vi "Acquire Finite Frames.vi"(8 "error in (no error)":errorcluster, 11 "TroSpec in":refnum<class "PL ISTEQ TroSpec.lvclass">) -> (0 "error out":errorcluster, 1 "lost frames":u16, 2 "frame":u32[][](array[numeric]), 3 "TroSpec out":refnum<class "PL ISTEQ TroSpec.lvclass">)   [LabVIEW 2015, in "PL ISTEQ TroSpec.lvclass"]
doc: "Starts acquisition and reads the configured finite number of frames."
uses:
  PL ISTEQ TroSpec.lvclass
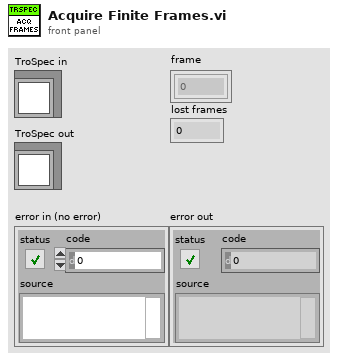
[diagram p1: front panel]
types:
  T1 = cluster{"period, s":dbl, "gain":u16, "offset":u16, "mode":cluster{"acquisition":bool, "service mode":bool, "inverted X":bool, "continuous acquisition":bool, "multiple exposures":bool}, "number of frames":u32, "exposure":u32}
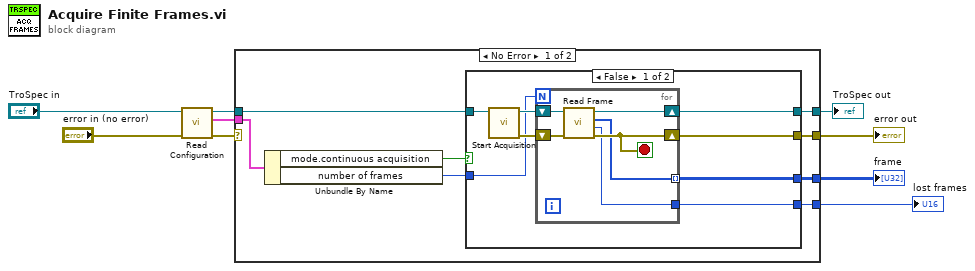
[diagram p0: block diagram]
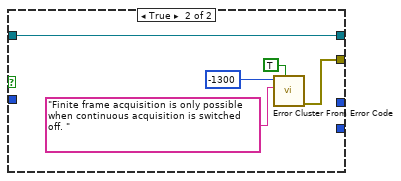
[diagram p2: hidden frame]
diagram:
  n1 = call "Read Configuration.vi"("error in (no error)"="error in (no error)", "TroSpec in"="TroSpec in") -> ("error out"=w7:errorcluster, "configuration"=w3:T1, "TroSpec out"=w6:refnum<class "PL ISTEQ TroSpec.lvclass">)  [unwired: 7 in]
  n2 = case shown="No Error" w7 {
    selector: w7 -> [_ w37]
    tunnel: w6 -> [w14 w38]
    tunnel: [w13 w38] -> w5
    tunnel: [w15 w37] -> w4
    tunnel: w3 -> [w17 _]
    tunnel: [w12 _] -> w2
    tunnel: [w11 _] -> w1
    frame No Error {
      n3 = Unbundle By Name(w17) -> ("mode.continuous acquisition"=w16:bool, "number of frames"=w10:u32)
      n4 = case shown="False" w16 {
        tunnel: [w22 w33] -> w15
        tunnel: w14 -> [w25 w32]
        tunnel: [w21 w32] -> w13
        tunnel: [w20 _] -> w12
        tunnel: [w19 _] -> w11
        tunnel: w10 -> [w18 _]
        frame False {
          n5 = call "Start Acquisition.vi"("TroSpec in"=w25) -> ("error out"=w23:errorcluster, "TroSpec out"=w24:refnum<class "PL ISTEQ TroSpec.lvclass">)  [unwired: 9 in]
          n6 = for {
            N: w18 -> [_]
            shift-right: [w26] -> w21
            shift-left: w24 -> [w31]
            shift-right: [w29] -> w22
            shift-left: w23 -> [w30]
            tunnel: [w28] -> w19
            tunnel: [w27] -> w20 mode=indexing
            stop <- w29 stop-if-true
            n7 = call "Read Frame.vi"("error in (no error)"=w30, "TroSpec in"=w31) -> ("error out"=w29:errorcluster, "lost frames"=w28:u16, "frame"=w27:u32[], "TroSpec out"=w26:refnum<class "PL ISTEQ TroSpec.lvclass">)  [unwired: 6 in]
          }
        }
        frame True {
          n8 = call <vilib>:"Error Cluster From Error Code.vi"("show call chain? (False)"=TRUE, "error message (\"\")"="Finite frame acquisition is only possible when continuous acquisition is switched off. " ("format string"), "error code (0)"=-1300) -> ("error out"=w33:errorcluster)  [unwired: 6 in]
        }
      }
    }
    frame Error {
    }
  }
  "error out" <- w4
  "TroSpec out" <- w5
  "frame" <- w2
  "lost frames" <- w1
